vi "getCorrectData.vi"(0 "reference in":refnum<class "excelFile.lvclass">, 1 "Refnum Cluster In":T1, 2 "Start":cluster{"Column":i32, "Row":i32}, 3 "End":cluster{"Column":i32, "Row":i32}, 5 "error in (no error)":errorcluster) -> (14 "reference out":refnum<class "excelFile.lvclass">, 15 "Refnum Cluster Out":T1, 16 "data":string[][](array[string]), 19 "error out":errorcluster)   [LabVIEW 2015, in "excelFile.lvclass"]
uses:
  excelFile.lvclass
  <userlib>/Read_Excel_Values.llb/GetXL_CellValues_2D_String.vi
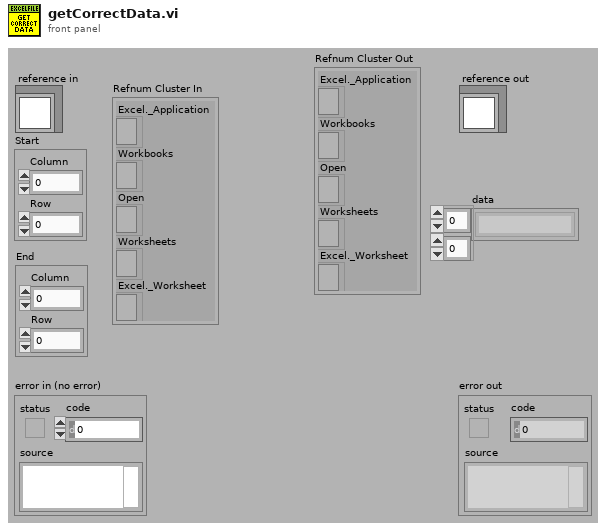
[diagram p1: front panel]
types:
  T1 = cluster{"Excel._Application":refnum<k7>, "Workbooks":refnum<k7>, "Open":refnum<k7>, "Worksheets":refnum<k7>, "Excel._Worksheet":refnum<k7>}
  T2 = typedef "excelFile.lvclass/ObjectAttributesRef.ctl" = refnum<data-value>
  T3 = typedef "excelFile.lvclass/ObjectAttributes.ctl" = cluster{"MyAttribute":dbl, "path":string, "Refnum Excel":cluster{"Excel._Application":refnum<k7>, "Workbooks":refnum<k7>, "Open":refnum<k7>}, "data":string[][][], "fileType":T4, "sheetName":string[]}
  T4 = typedef "excelFile.lvclass/fileType.ctl" = enum16{"database", "CosmedTest PFTSUITE", "CosmedTest OMNIA"}
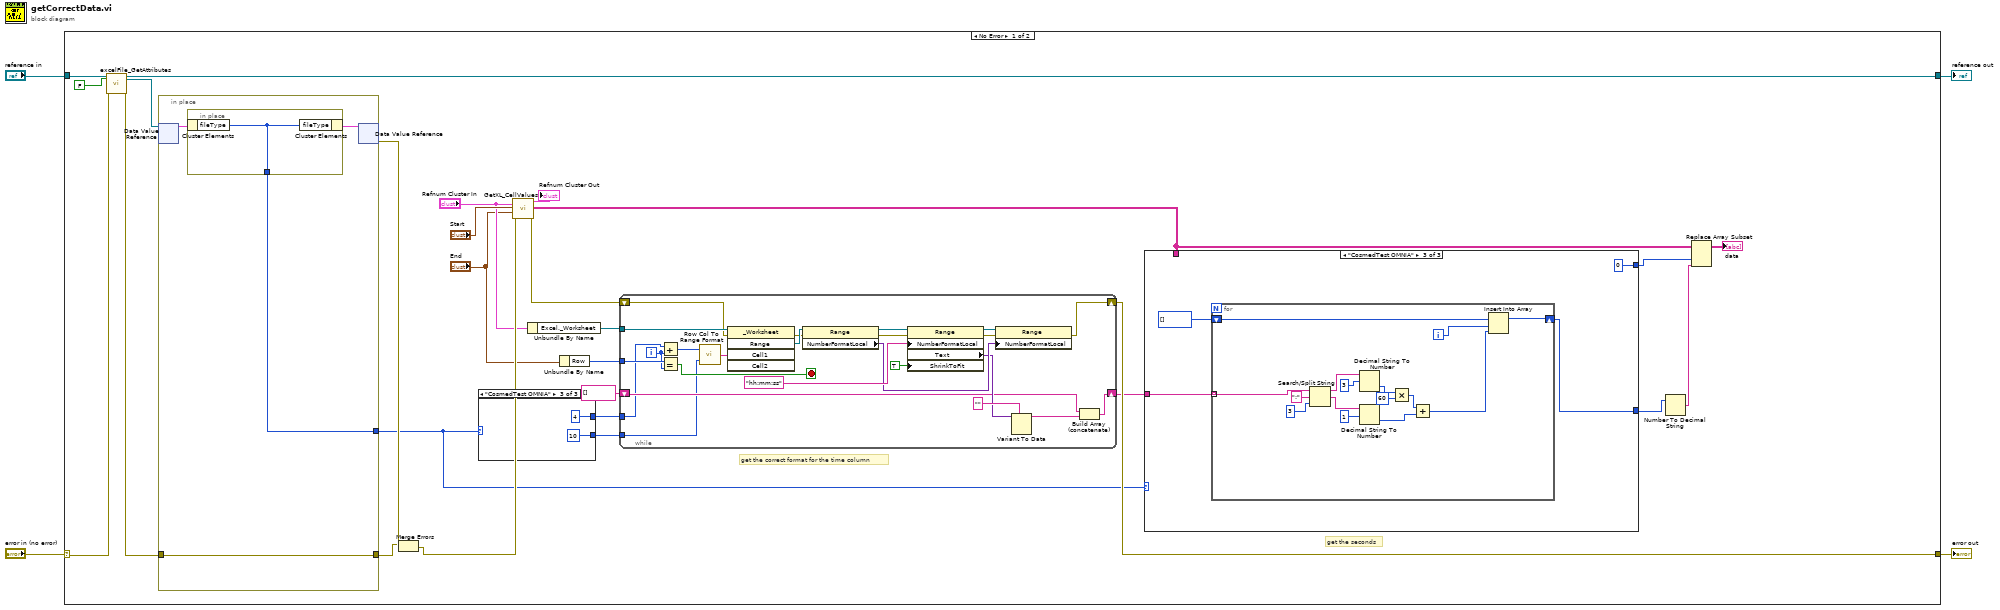
[diagram p0: block diagram]
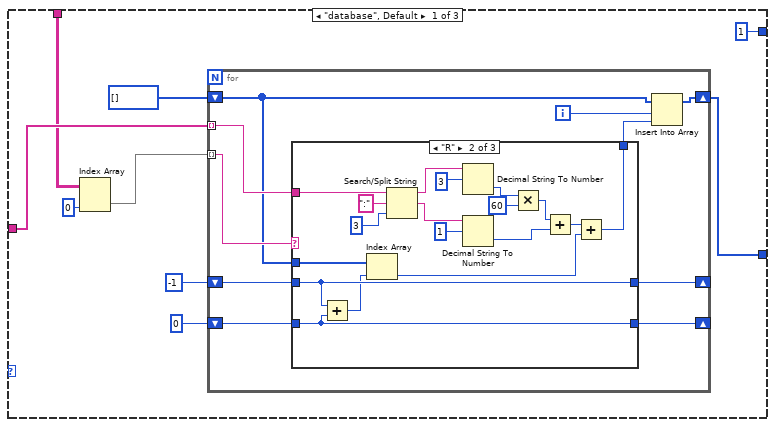
[diagram p2: hidden frame]
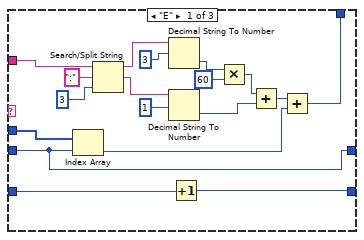
[diagram p3: hidden frame]
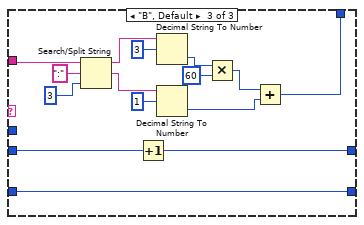
[diagram p4: hidden frame]
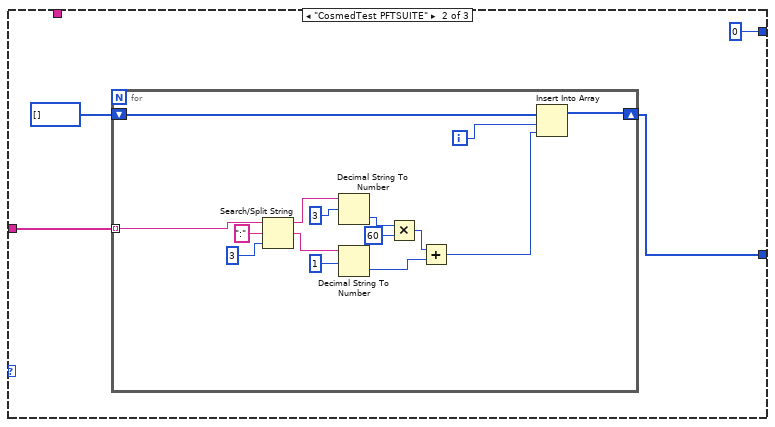
[diagram p5: hidden frame]
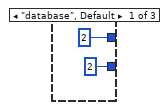
[diagram p6: hidden frame]
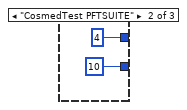
[diagram p7: hidden frame]
diagram:
  n1 = case shown="No Error" "error in (no error)" {
    selector: "error in (no error)" -> [w27 w176]
    tunnel: [w20 w176] -> w3
    tunnel: [w25 w175] -> w1
    tunnel: "reference in" -> [w29 w175]
    frame No Error {
      # "get the seconds"
      # "get the correct format for the time column"
      n2 = call "excelFile_GetAttributes.vi"("reference in"=w29, "return data? (T)"=FALSE, "error in (no error)"=w27) -> ("reference out"=w25:refnum<class "excelFile.lvclass">, "attributes ref"=w24:T2, "error out"=w26:errorcluster)  [unwired: 13 in, 1 out]
      n3 = in-place {
        in-place-border: w26 -> [w171]
        in-place-border: [w171] -> w30
        in-place-border: [w170] -> w11
        n4 = in-place-dvr #1(w24) -> (w172:T3)  [unwired: 1 out]
        n5 = in-place {
          in-place-border: [w174] -> w170
          n6 = in-place-cluster #2(w172) -> ("fileType"=w174:T4)
          n7 = in-place-cluster #2("fileType"=w174) -> (w173:T3)
        }
        n8 = in-place-dvr #1(w173) -> (w31:errorcluster)  [unwired: 1 out]
      }
      n9 = Merge Errors(w30, w31) -> (w23:errorcluster)
      n10 = case shown="\"CosmedTest OMNIA\"" w11 {
        tunnel: [2 10 10] -> w14
        tunnel: [2 4 4] -> w13
        frame "database", Default {
        }
        frame "CosmedTest PFTSUITE" {
        }
        frame "CosmedTest OMNIA" {
        }
      }
      n11 = call-poly <userlib>:"GetXL_CellValues.vi"("error in"=w23, "End"="End", "Start"="Start", "Refnum Cluster In"="Refnum Cluster In") -> ("error out"=w21:errorcluster, "data"=w8:string[][], "Refnum Cluster Out"=→"Refnum Cluster Out":T1)  [unwired: 5 in]
      n12 = Unbundle By Name("Refnum Cluster In") -> ("Excel._Worksheet"=w17:refnum<k7>)
      n13 = Unbundle By Name("End") -> ("Row"=w15:i32)
      n14 = while {
        tunnel: w17 -> [w163]
        shift-right: [w156] -> w12
        shift-left: string[] [] -> [w158]
        tunnel: w15 -> [w155]
        shift-right: [w149] -> w20
        shift-left: w21 -> [w148]
        tunnel: w14 -> [w147]
        tunnel: w13 -> [w146]
        i -> [w152]
        stop <- w154 stop-if-true
        n15 = Add(x=w146, y=w152) -> (x+y=w151:i32)
        n16 = Equal?(x=w155, y=w152) -> (x = y?=w154:bool)
        n17 = call <userlib>:"Row Col To Range Format.vi"("Column"=w147, "Row"=w151) -> ("Output String"=w153:string)
        n18 = invoke class="_Worksheet" method="Range"(reference=w163, error in=w148, "Cell1"=w153) -> (error out=w167:errorcluster, "Range"=w169:refnum<k7>)  [unwired: 2 in, 3 out]
        n19 = property class="Range"(reference=w169, error in=w167) -> (reference out=w168:refnum<k7>, error out=w166:errorcluster, "NumberFormatLocal"=w164:variant)
        n20 = property class="Range"(reference=w168, error in=w166, "NumberFormatLocal"="hh:mm:ss" ("data 3"), "ShrinkToFit"=TRUE) -> (reference out=w160:refnum<k7>, error out=w150:errorcluster, "Text"=w161:variant)
        n21 = property class="Range"(reference=w160, error in=w150, "NumberFormatLocal"=w164) -> (error out=w149:errorcluster)  [unwired: 1 out]
        n22 = Variant To Data(type="", Variant=w161) -> (data=w157:string)  [unwired: 1 in, 1 out]
        n23 = Build Array (concatenate)(w158, w157) -> (w156:string[])
      }
      n24 = case shown="\"CosmedTest OMNIA\"" w11 {
        tunnel: w12 -> [w35 w105 w124]
        tunnel: w8 -> [w34 _ _]
        tunnel: [w33 w102 w121] -> w10
        tunnel: [1 ("disabled index (col)") 0 ("disabled index (col)") 0 ("disabled index (col)")] -> w7
        frame "database", Default {
          n25 = Index Array(array=w34, index (col)=0 ("disabled index (col)")) -> (element=w38:string[])  [unwired: 1 in]
          n26 = for {
            tunnel: w35 -> [w49] mode=indexing
            shift-right: [w48] -> w33
            shift-left: i32[] [] -> [w44]
            tunnel: w38 -> [w50] mode=indexing
            shift-right: [w45] -> _
            shift-left: -1 -> [w42]
            shift-right: [w43] -> _
            shift-left: 0 -> [w41]
            i -> [w47]
            n27 = case shown="\"R\"" w50 {
              tunnel: w49 -> [w60 w75 w101]
              tunnel: [w54 w74 w92] -> w46
              tunnel: w42 -> [w51 w70 w91]
              tunnel: [w51 w70 w90] -> w45
              tunnel: w44 -> [w58 w76 _]
              tunnel: w41 -> [w56 w71 w89]
              tunnel: [w55 w71 w89] -> w43
              frame "E" {
                n28 = Index Array(array=w58, index=w51) -> (element=w57:i32)
                n29 = Search/Split String(string=w60, search string/char (-)=":", offset (0)=3) -> (substring before match=w66:string, match + rest of string=w65:string)  [unwired: 1 out]
                n30 = Decimal String To Number(string=w66, offset=3) -> (number=w64:i32)  [unwired: 1 in, 1 out]
                n31 = Decimal String To Number(string=w65, offset=1) -> (number=w61:i32)  [unwired: 1 in, 1 out]
                n32 = Increment(x=w56) -> (x+1=w55:i32)
                n33 = Multiply(x=w64, y=60) -> (x*y=w62:i32)
                n34 = Add(x=w62, y=w61) -> (x+y=w59:i32)
                n35 = Add(x=w59, y=w57) -> (x+y=w54:i32)
              }
              frame "R" {
                n36 = Add(x=w70, y=w71) -> (x+y=w69:i32)
                n37 = Index Array(array=w76, index=w69) -> (element=w77:i32)
                n38 = Search/Split String(string=w75, search string/char (-)=":", offset (0)=3) -> (substring before match=w84:string, match + rest of string=w83:string)  [unwired: 1 out]
                n39 = Decimal String To Number(string=w84, offset=3) -> (number=w82:i32)  [unwired: 1 in, 1 out]
                n40 = Decimal String To Number(string=w83, offset=1) -> (number=w79:i32)  [unwired: 1 in, 1 out]
                n41 = Multiply(x=w82, y=60) -> (x*y=w80:i32)
                n42 = Add(x=w80, y=w79) -> (x+y=w78:i32)
                n43 = Add(x=w78, y=w77) -> (x+y=w74:i32)
              }
              frame "B", Default {
                n44 = Search/Split String(string=w101, search string/char (-)=":", offset (0)=3) -> (substring before match=w98:string, match + rest of string=w97:string)  [unwired: 1 out]
                n45 = Increment(x=w91) -> (x+1=w90:i32)
                n46 = Decimal String To Number(string=w98, offset=3) -> (number=w96:i32)  [unwired: 1 in, 1 out]
                n47 = Decimal String To Number(string=w97, offset=1) -> (number=w93:i32)  [unwired: 1 in, 1 out]
                n48 = Multiply(x=w96, y=60) -> (x*y=w94:i32)
                n49 = Add(x=w94, y=w93) -> (x+y=w92:i32)
              }
            }
            n50 = Insert Into Array(array=w44, index=w47, new element=w46) -> (w48:i32[])
          }
        }
        frame "CosmedTest PFTSUITE" {
          n51 = for {
            tunnel: w105 -> [w110] mode=indexing
            shift-right: [w108] -> w102
            shift-left: i32[] [] -> [w109]
            i -> [w106]
            n52 = Search/Split String(string=w110, search string/char (-)=":", offset (0)=3) -> (substring before match=w113:string, match + rest of string=w114:string)  [unwired: 1 out]
            n53 = Decimal String To Number(string=w113, offset=3) -> (number=w115:i32)  [unwired: 1 in, 1 out]
            n54 = Decimal String To Number(string=w114, offset=1) -> (number=w118:i32)  [unwired: 1 in, 1 out]
            n55 = Multiply(x=w115, y=60) -> (x*y=w117:i32)
            n56 = Add(x=w117, y=w118) -> (x+y=w107:i32)
            n57 = Insert Into Array(array=w109, index=w106, new element=w107) -> (w108:i32[])
          }
        }
        frame "CosmedTest OMNIA" {
          n58 = for {
            tunnel: w124 -> [w129] mode=indexing
            shift-right: [w127] -> w121
            shift-left: i32[] [] -> [w128]
            i -> [w125]
            n59 = Search/Split String(string=w129, search string/char (-)=":", offset (0)=3) -> (substring before match=w132:string, match + rest of string=w133:string)  [unwired: 1 out]
            n60 = Decimal String To Number(string=w132, offset=3) -> (number=w134:i32)  [unwired: 1 in, 1 out]
            n61 = Decimal String To Number(string=w133, offset=1) -> (number=w137:i32)  [unwired: 1 in, 1 out]
            n62 = Multiply(x=w134, y=60) -> (x*y=w136:i32)
            n63 = Add(x=w136, y=w137) -> (x+y=w126:i32)
            n64 = Insert Into Array(array=w128, index=w125, new element=w126) -> (w127:i32[])
          }
        }
      }
      n65 = Number To Decimal String(number=w10) -> (decimal integer string=w9:string[])  [unwired: 1 in]
      n66 = Replace Array Subset(array=w8, new element=w9, index (col)=w7) -> (→"data":string[][])  [unwired: 1 in]
    }
    frame Error {
    }
  }
  "error out" <- w3
  "reference out" <- w1
